vi "Naming Check.vi"(8 "error in (no error)":errorcluster, 11 "Name(\"\" to use uuid)":string) -> (0 "error out":errorcluster, 3 "Name(dup)":string)   [LabVIEW 2014, in "JKI State Machine++.lvlib"]
uses:
  JKI State Machine++.lvlib
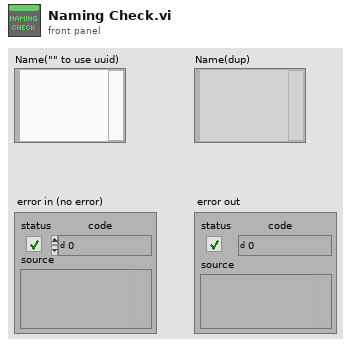
[diagram p1: front panel]
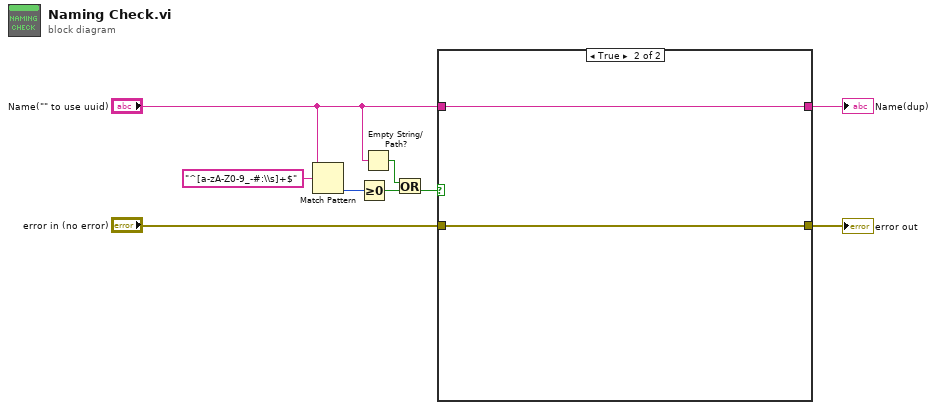
[diagram p0: block diagram]
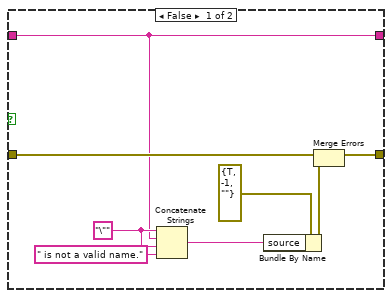
[diagram p2: hidden frame]
diagram:
  n1 = Match Pattern(string="Name(\"\" to use uuid)", regular expression="^[a-zA-Z0-9_-#:\\s]+$") -> (offset past match=w6:i32)  [unwired: 1 in, 3 out]
  n2 = Greater Or Equal To 0?(x=w6) -> (x >= 0?=w5:bool)
  n3 = Empty String/Path?(string/path="Name(\"\" to use uuid)") -> (empty?=w1:bool)
  n4 = Or(x=w1, y=w5) -> (x .or. y?=w2:bool)
  n5 = case shown="True" w2 {
    tunnel: "error in (no error)" -> [w17 w19]
    tunnel: [w16 w19] -> w8
    tunnel: [w13 w18] -> w4
    tunnel: "Name(\"\" to use uuid)" -> [w13 w18]
    frame False {
      w14 = "\"" ("string")
      n6 = Concatenate Strings(w14, w13, w14, " is not a valid name." ("string")) -> (w10:string)
      n7 = Bundle By Name(cluster=errorcluster {"status"=TRUE, "code"=-1, "source"=""} ("error in"), "source"=w10) -> (w11:errorcluster)
      n8 = Merge Errors(w17, w11) -> (w16:errorcluster)
    }
    frame True {
    }
  }
  "error out" <- w8
  "Name(dup)" <- w4
